vi "Default Settings.vi"(8 "error in (no error)":errorcluster, 10 "Module In":refnum<class "Module.lvclass">, 11 "Carrier Tray in":refnum<class "Assembly Tray.lvclass">) -> (0 "error out":errorcluster, 2 "Module Out":refnum<class "Module.lvclass">, 3 "Carrier Tray out":refnum<class "Assembly Tray.lvclass">)   [LabVIEW 2016, in "Assembly Tray.lvclass"]
uses:
  Assembly Tray.lvclass
  C:/Users/HEP Gantry/Documents/Assembly/V5/Classes/Workspace/Fixture.lvclass
  Module/Module.lvclass
  Module/Module.lvclass/Module.ctl
  Fixture.lvclass/Fixture.ctl
  Assembly Tray.lvclass/Assembly Tray.ctl
  Module/Read Tray Number.vi
  Module/Read Tray Position.vi
  Module/Read Tray Region.vi
  Module/Read Module Thickness.vi
  Write Gantry Region.vi
  Write Fixture ID.vi
  Write Position.vi
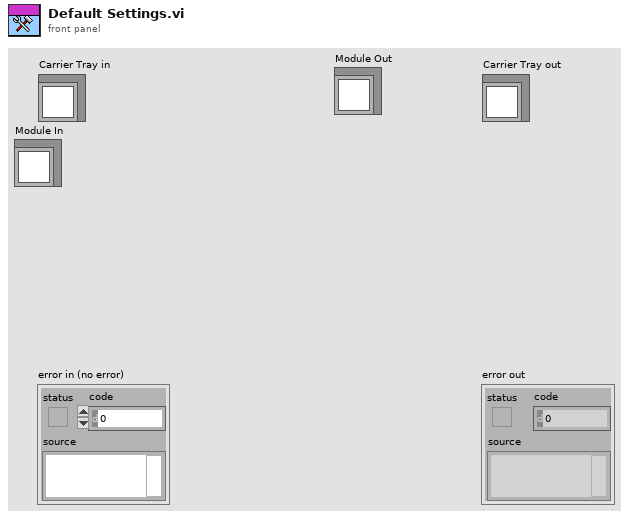
[diagram p1: front panel]
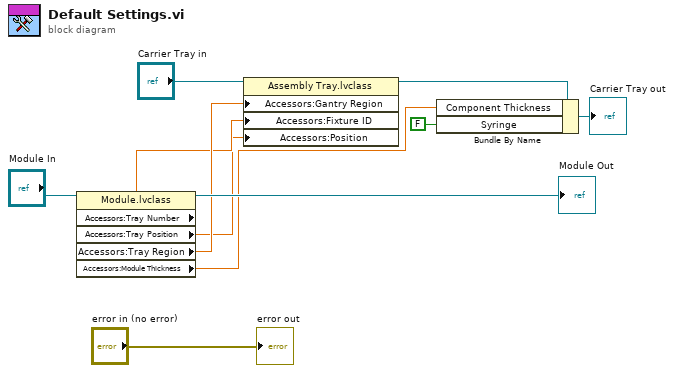
[diagram p0: block diagram]
diagram:
  n1 = property class="Module.lvclass"(reference="Module In") -> (reference out=→"Module Out":refnum<class "Module.lvclass">, "Accessors:Tray Number"=w3:dbl, "Accessors:Tray Position"=w2:dbl, "Accessors:Tray Region"=w6:dbl, "Accessors:Module Thickness"=w5:dbl)  [unwired: 1 in, 1 out]
  n2 = property class="Assembly Tray.lvclass"(reference="Carrier Tray in", "Accessors:Gantry Region"=w6, "Accessors:Fixture ID"=w3, "Accessors:Position"=w2) -> (reference out=w9:refnum<class "Assembly Tray.lvclass">)  [unwired: 1 in, 1 out]
  n3 = Bundle By Name(cluster=w9, "Component Thickness"=w5, "Syringe"=FALSE) -> (→"Carrier Tray out":refnum<class "Assembly Tray.lvclass">)
  "error out" <- "error in (no error)"
